vi "Get Package Dependencies.vi"(8 "error in":errorcluster, 10 "version":string, 11 "package name":string) -> (0 "error out":errorcluster, 3 "package dependencies":string[][](table))   [LabVIEW 2014, in "NIPM_API.lvlib"]
doc: "Get the full package dependency tree for the given package. The list does include the specified package.\n\nINPUT(s)\n<B>Package name</B>: Specifies the package\n<B>Version</B>: Specifies the package version\n\nOUTPUT(s)\n<B>Installed packages</B>: Outputs a list of dependent packages and their versions"
uses:
  NIPM_API.lvlib
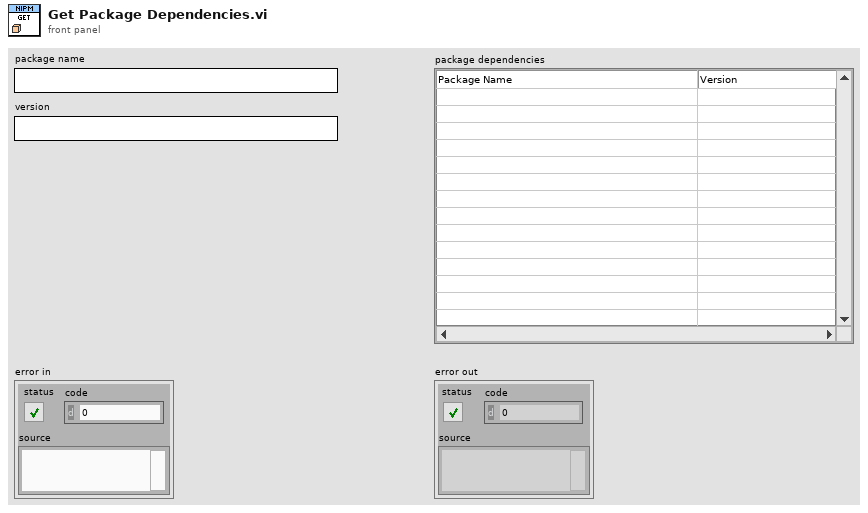
[diagram p1: front panel]
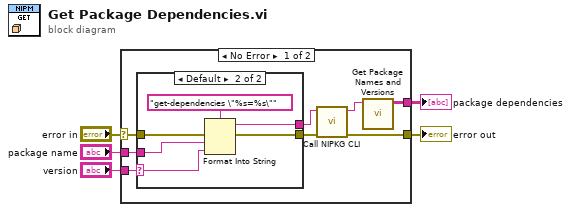
[diagram p0: block diagram]
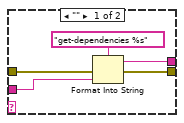
[diagram p2: hidden frame]
diagram:
  n1 = case shown="No Error" "error in" {
    selector: "error in" -> [w12 w25]
    tunnel: [w13 w25] -> w4
    tunnel: [w10 _] -> w5
    tunnel: "package name" -> [w6 _]
    tunnel: "version" -> [w7 _]
    frame No Error {
      n2 = case shown="Default" w7 {
        selector: w7 -> [_ w19]
        tunnel: w12 -> [w18 w24]
        tunnel: [w17 w23] -> w9
        tunnel: [w16 w22] -> w8
        tunnel: w6 -> [w15 w21]
        frame "" {
          n3 = Format Into String(format string="get-dependencies %s", error in=w18, w15) -> (resulting string=w16:string, error out=w17:errorcluster)  [unwired: 1 in]
        }
        frame Default {
          n4 = Format Into String(format string="get-dependencies \"%s=%s\"", error in=w24, w21, w19) -> (resulting string=w22:string, error out=w23:errorcluster)  [unwired: 1 in]
        }
      }
      n5 = call "Call NIPKG CLI.vi"("error in (no error)"=w9, "command"=w8) -> ("error out"=w13:errorcluster, "command line standard output"=w11:string)  [unwired: 8 in]
      n6 = call "Get Package Names and Versions.vi"("NIPKG Result"=w11) -> ("Packages"=w10:string[][])  [unwired: 10 in]
    }
    frame Error {
    }
  }
  "package dependencies" <- w5
  "error out" <- w4
